vi "EnumDevicesEx2.vi"(5 "nLayerType":u32=1, 11 "error in (no error)":errorcluster caption="错误输入（无错误）") -> (4 "function return":i32, 6 "nDeviceNumReturn":u32, 8 "GigEDeviceArray":T4(array[cluster]), 10 "U3VDeviceArray":T3(array[cluster]), 12 "GenTLDevice":T1(array[cluster]), 15 "error out":errorcluster caption="错误输出")   [LabVIEW 2013, in "MvCameraControl.lvlib"]
uses:
  MvCameraControl.lvlib
  MvCameraPatch.dll
panel:
  in  "enSortMethod":T2(ring)
  in  "strManufacturerName":i8[](array[numeric])
  in  "U3VDevice":T5
  in  "GigEDevice":T6
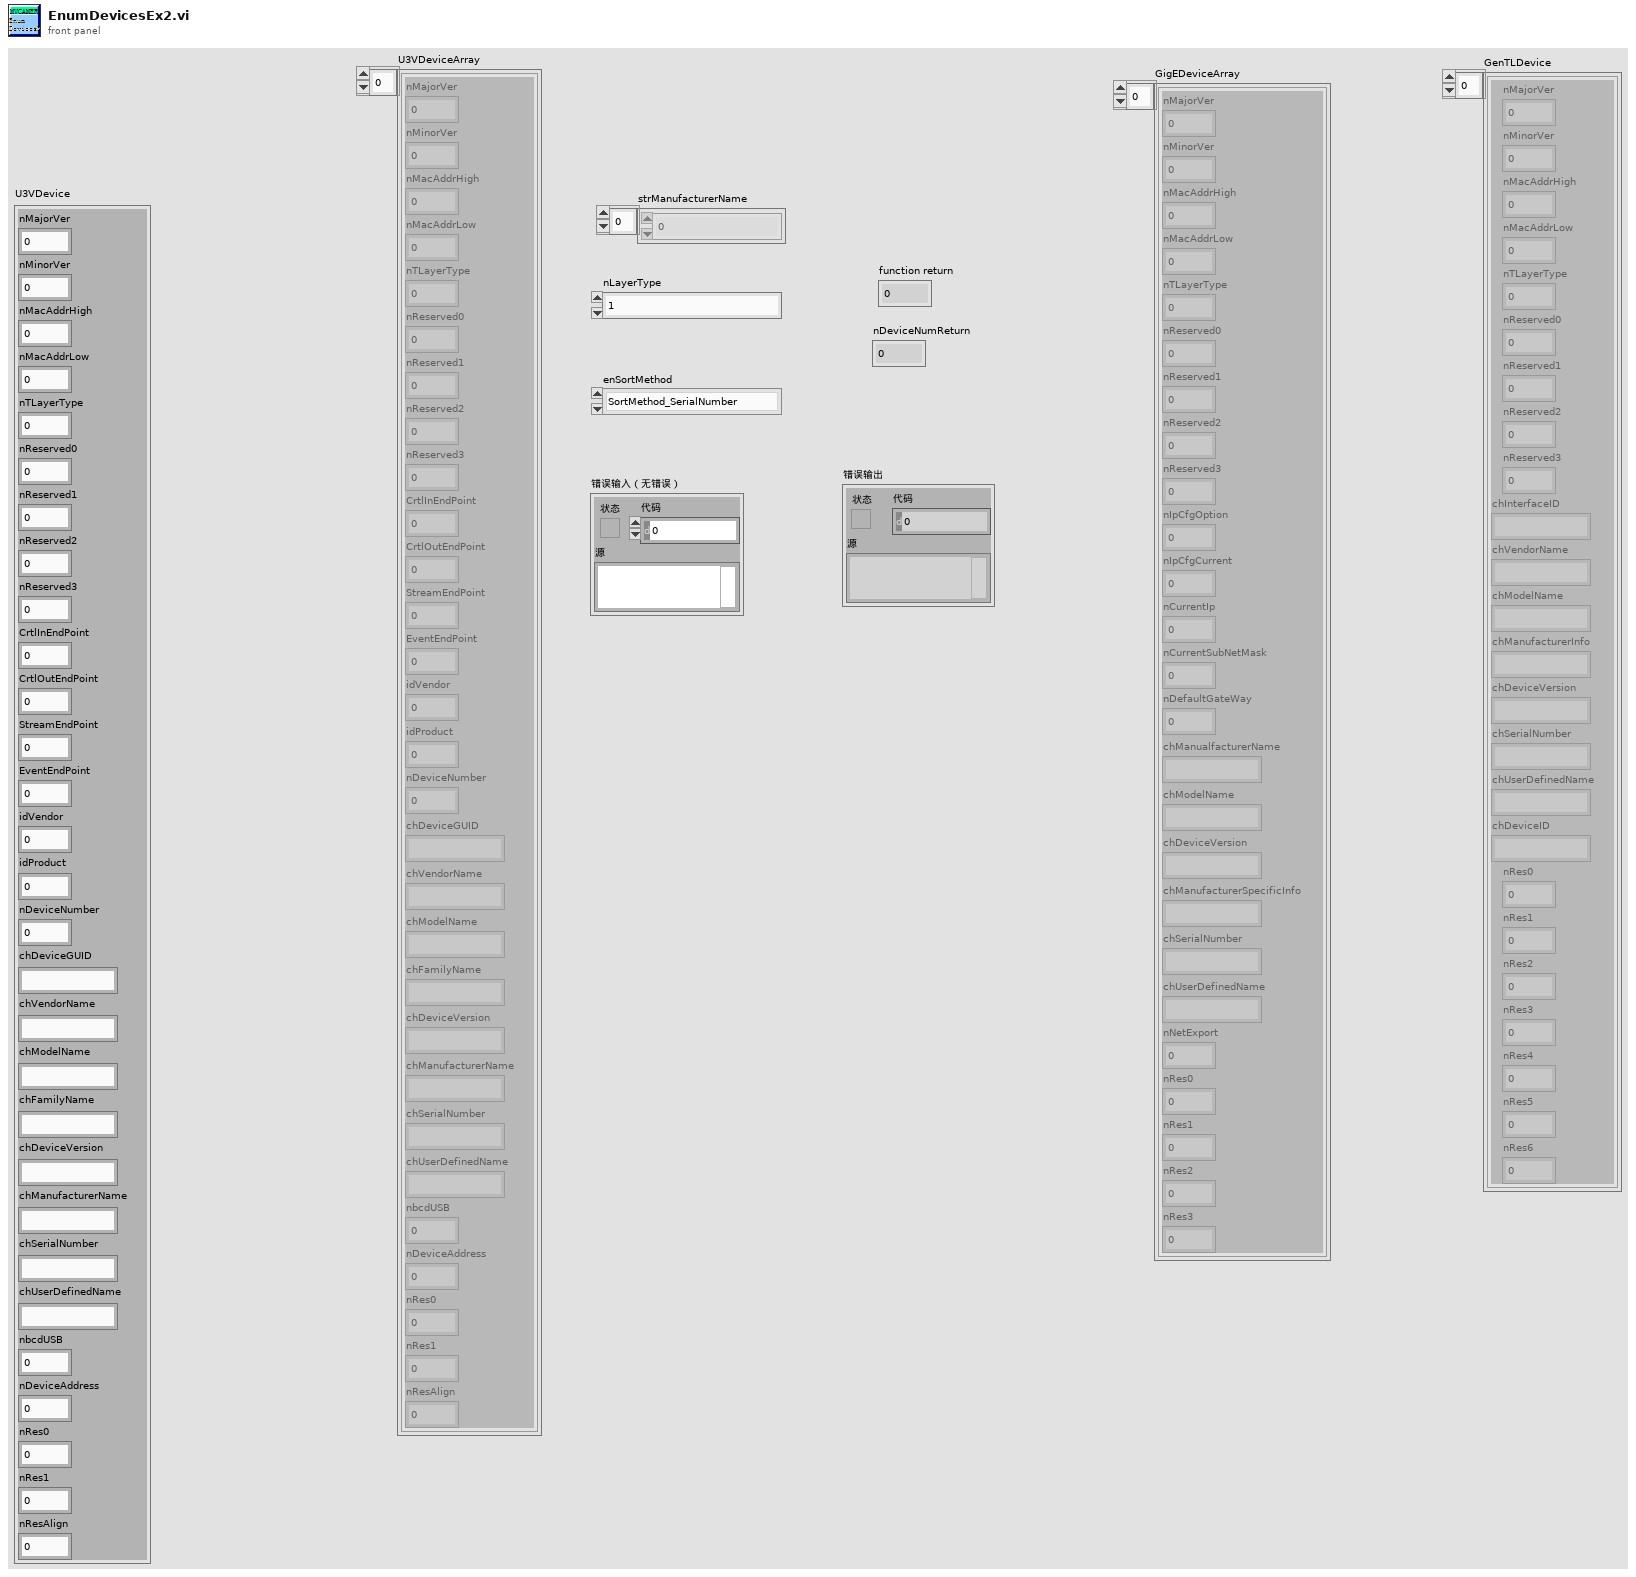
[diagram p1: front panel]
types:
  T1 = cluster{"nMajorVer":u16, "nMinorVer":u16, "nMacAddrHigh":u32, "nMacAddrLow":u32, "nTLayerType":u32, "nReserved0":u32, "nReserved1":u32, "nReserved2":u32, "nReserved3":u32, "chInterfaceID":string, "chVendorName":string, "chModelName":string, "chManufacturerInfo":string, "chDeviceVersion":string, "chSerialNumber":string, "chUserDefinedName":string, "chDeviceID":string, "nRes0":u32, "nRes1":u32, "nRes2":u32, "nRes3":u32, "nRes4":u32, "nRes5":u32, "nRes6":u32}[]
  T2 = enum16{"SortMethod_SerialNumber", "SortMethod_UserID", "SortMethod_CurrentIP_ASC", "SortMethod_CurrentIP_DESC"}
  T3 = cluster{"nMajorVer":u16, "nMinorVer":u16, "nMacAddrHigh":u32, "nMacAddrLow":u32, "nTLayerType":u32, "nReserved0":u32, "nReserved1":u32, "nReserved2":u32, "nReserved3":u32, "CrtlInEndPoint":u8, "CrtlOutEndPoint":u8, "StreamEndPoint":u8, "EventEndPoint":u8, "idVendor":u16, "idProduct":u16, "nDeviceNumber":u32, "chDeviceGUID":string, "chVendorName":string, "chModelName":string, "chFamilyName":string, "chDeviceVersion":string, "chManufacturerName":string, "chSerialNumber":string, "chUserDefinedName":string, "nbcdUSB":u32, "nDeviceAddress":u32, "nRes0":u32, "nRes1":u32, "nResAlign":u32}[]
  T4 = cluster{"nMajorVer":u16, "nMinorVer":u16, "nMacAddrHigh":u32, "nMacAddrLow":u32, "nTLayerType":u32, "nReserved0":u32, "nReserved1":u32, "nReserved2":u32, "nReserved3":u32, "nIpCfgOption":u32, "nIpCfgCurrent":u32, "nCurrentIp":u32, "nCurrentSubNetMask":u32, "nDefaultGateWay":u32, "chManualfacturerName":string, "chModelName":string, "chDeviceVersion":string, "chManufacturerSpecificInfo":string, "chSerialNumber":string, "chUserDefinedName":string, "nNetExport":u32, "nRes0":u32, "nRes1":u32, "nRes2":u32, "nRes3":u32}[]
  T5 = cluster{"nMajorVer":u16, "nMinorVer":u16, "nMacAddrHigh":u32, "nMacAddrLow":u32, "nTLayerType":u32, "nReserved0":u32, "nReserved1":u32, "nReserved2":u32, "nReserved3":u32, "CrtlInEndPoint":u8, "CrtlOutEndPoint":u8, "StreamEndPoint":u8, "EventEndPoint":u8, "idVendor":u16, "idProduct":u16, "nDeviceNumber":u32, "chDeviceGUID":string, "chVendorName":string, "chModelName":string, "chFamilyName":string, "chDeviceVersion":string, "chManufacturerName":string, "chSerialNumber":string, "chUserDefinedName":string, "nbcdUSB":u32, "nDeviceAddress":u32, "nRes0":u32, "nRes1":u32, "nResAlign":u32}
  T6 = cluster{"nMajorVer":u16, "nMinorVer":u16, "nMacAddrHigh":u32, "nMacAddrLow":u32, "nTLayerType":u32, "nReserved0":u32, "nReserved1":u32, "nReserved2":u32, "nReserved3":u32, "nIpCfgOption":u32, "nIpCfgCurrent":u32, "nCurrentIp":u32, "nCurrentSubNetMask":u32, "nDefaultGateWay":u32, "chManualfacturerName":string, "chModelName":string, "chDeviceVersion":string, "chManufacturerSpecificInfo":string, "chSerialNumber":string, "chUserDefinedName":string, "nNetExport":u32, "nRes0":u32, "nRes1":u32, "nRes2":u32, "nRes3":u32}
  T7 = cluster{"nMajorVer":u16, "nMinorVer":u16, "nMacAddrHigh":u32, "nMacAddrLow":u32, "nTLayerType":u32, "nReserved0":u32, "nReserved1":u32, "nReserved2":u32, "nReserved3":u32, "chInterfaceID":string, "chVendorName":string, "chModelName":string, "chManufacturerInfo":string, "chDeviceVersion":string, "chSerialNumber":string, "chUserDefinedName":string, "chDeviceID":string, "nRes0":u32, "nRes1":u32, "nRes2":u32, "nRes3":u32, "nRes4":u32, "nRes5":u32, "nRes6":u32}
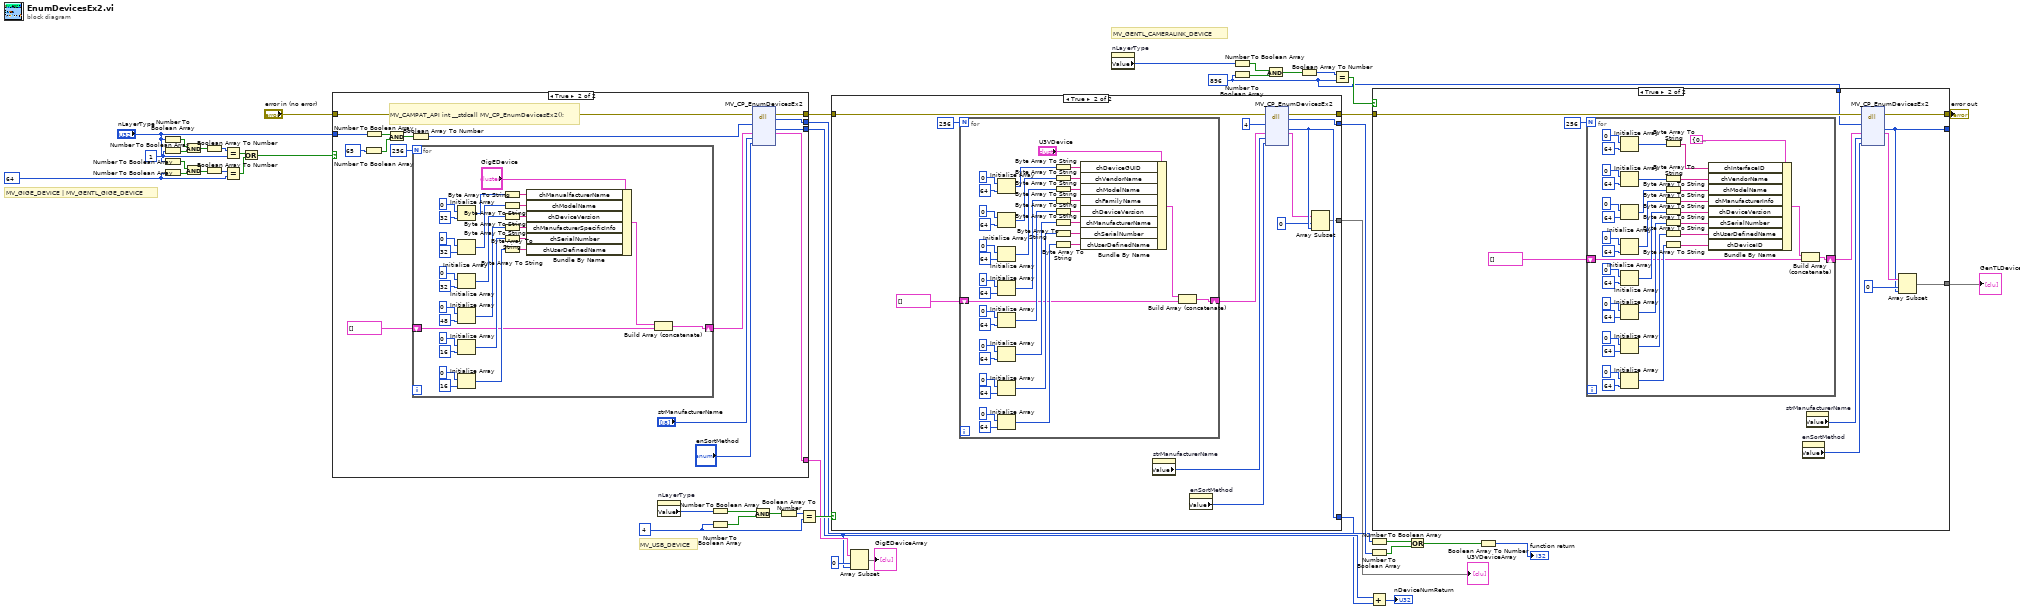
[diagram p0: block diagram]
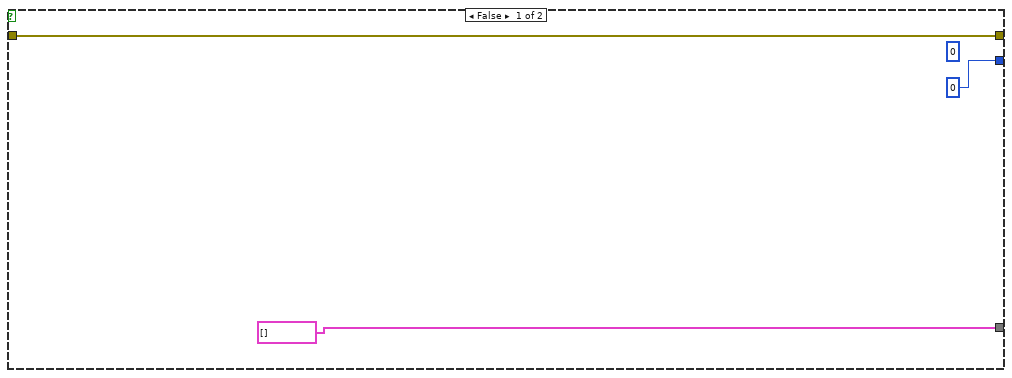
[diagram p2: hidden frame]
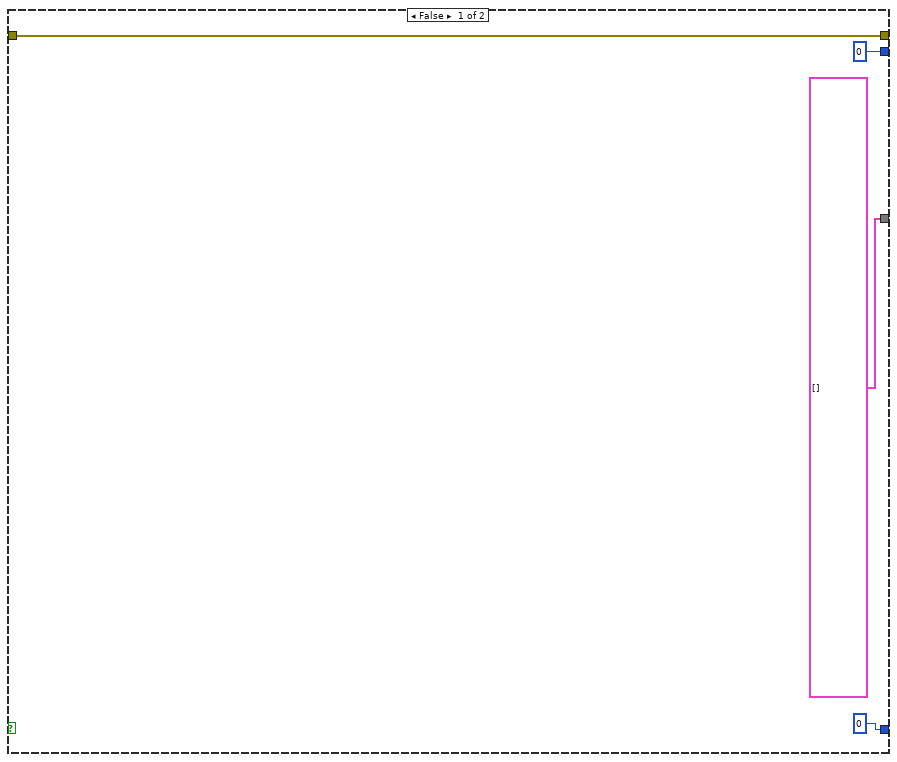
[diagram p3: hidden frame]
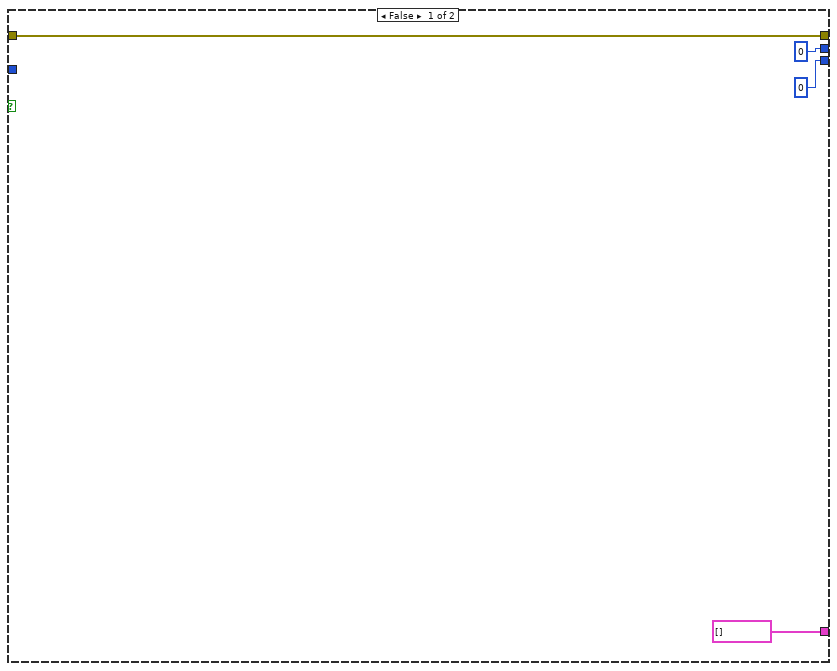
[diagram p4: hidden frame]
diagram:
  w2 = u32 896 ("数字")
  w17 = u32 64 ("数字")
  w36 = u32 4 ("数字")
  w42 = u32 1 ("数字")
  # "MV_GENTL_CAMERALINK_DEVICE"
  # "MV_USB_DEVICE"
  # "MV_GIGE_DEVICE | MV_GENTL_GIGE_DEVICE"
  n1 = Number To Boolean Array(number="nLayerType") -> (Boolean array=w46:bool[])
  n2 = Number To Boolean Array(number=w42) -> (Boolean array=w45:bool[])
  n3 = Number To Boolean Array(number="nLayerType") -> (Boolean array=w21:bool[])
  n4 = Number To Boolean Array(number=w17) -> (Boolean array=w20:bool[])
  n5 = And(x=w46, y=w45) -> (x .and. y?=w44:bool[])
  n6 = And(x=w21, y=w20) -> (x .and. y?=w19:bool[])
  n7 = Boolean Array To Number(Boolean array=w44) -> (number=w43:u32)
  n8 = Boolean Array To Number(Boolean array=w19) -> (number=w18:u32)
  n9 = Equal?(x=w43, y=w42) -> (x = y?=w15:bool)
  n10 = Equal?(x=w18, y=w17) -> (x = y?=w16:bool)
  n11 = Or(x=w15, y=w16) -> (x .or. y?=w14:bool)
  n12 = case shown="True" w14 {
    tunnel: [0 ("返回类型") w64] -> w32
    tunnel: [u32 0 ("nDeviceNumReturn") w63] -> w24
    tunnel: "error in (no error)" -> [w48 w62]
    tunnel: [w48 w61] -> w27
    tunnel: [T4 [] ("DeviceInfoArray") w59] -> w26
    tunnel: "nLayerType" -> [_ w52]
    frame False {
    }
    frame True {
      # "MV_CAMPAT_API int __stdcall MV_CP_EnumDevicesEx2();"
      n13 = Number To Boolean Array(number=u32 65 ("数字")) -> (Boolean array=w55:bool[])
      n14 = Number To Boolean Array(number=w52) -> (Boolean array=w56:bool[])
      n15 = And(x=w56, y=w55) -> (x .and. y?=w54:bool[])
      n16 = Boolean Array To Number(Boolean array=w54) -> (number=w51:u32)
      n17 = for {
        N: 256 -> [_]
        shift-right: [w69] -> w66
        shift-left: T4 [] -> [w67]
        n18 = Initialize Array(u8 0 ("元素"), 32 ("维数大小")) -> (w78:u8[])
        n19 = Initialize Array(u8 0 ("元素"), 32 ("维数大小")) -> (w81:u8[])
        n20 = Initialize Array(u8 0 ("元素"), 32 ("维数大小")) -> (w70:u8[])
        n21 = Initialize Array(u8 0 ("元素"), 48 ("维数大小")) -> (w75:u8[])
        n22 = Initialize Array(u8 0 ("元素"), 16 ("维数大小")) -> (w89:u8[])
        n23 = Initialize Array(u8 0 ("元素"), 16 ("维数大小")) -> (w86:u8[])
        n24 = Byte Array To String(unsigned byte array=w78) -> (string=w90:string)
        n25 = Byte Array To String(unsigned byte array=w81) -> (string=w91:string)
        n26 = Byte Array To String(unsigned byte array=w70) -> (string=w71:string)
        n27 = Byte Array To String(unsigned byte array=w75) -> (string=w92:string)
        n28 = Byte Array To String(unsigned byte array=w89) -> (string=w93:string)
        n29 = Byte Array To String(unsigned byte array=w86) -> (string=w94:string)
        n30 = Bundle By Name(cluster="GigEDevice", "chManualfacturerName"=w90, "chModelName"=w91, "chDeviceVersion"=w71, "chManufacturerSpecificInfo"=w92, "chSerialNumber"=w93, "chUserDefinedName"=w94) -> (w68:T6)
        n31 = Build Array (concatenate)(w68, w67) -> (w69:T4)
      }
      n32 = dll-call lib="MvCameraPatch.dll" fn="MV_CP_EnumDevicesEx2"(error in=w62, "nLayerType"=w51, "DeviceInfoArray"=w66, "strManufacturerName"="strManufacturerName", "enSortMethod"="enSortMethod") -> (error out=w61:errorcluster, "返回类型"=w64:i32, "nDeviceNumReturn"=w63:u32, "DeviceInfoArray"=w59:T4)  [unwired: 6 in, 1 out]
    }
  }
  n33 = property on="nLayerType" class="DigNum (strict)"() -> ("Value"=w8:u32)  [unwired: 2 in, 2 out]
  n34 = Number To Boolean Array(number=w8) -> (Boolean array=w40:bool[])
  n35 = Number To Boolean Array(number=w36) -> (Boolean array=w39:bool[])
  n36 = And(x=w40, y=w39) -> (x .and. y?=w38:bool[])
  n37 = Boolean Array To Number(Boolean array=w38) -> (number=w37:u32)
  n38 = Equal?(x=w37, y=w36) -> (x = y?=w35:bool)
  n39 = case shown="True" w35 {
    tunnel: [u32 0 ("nDeviceNumReturn") w110] -> w22
    tunnel: [0 ("返回类型") w109] -> w33
    tunnel: w27 -> [w96 w108]
    tunnel: [w96 w107] -> w7
    tunnel: [T3 [] w99] -> w3
    frame False {
    }
    frame True {
      n40 = for {
        N: 256 -> [_]
        shift-right: [w112] -> w105
        shift-left: T3 [] -> [w114]
        n41 = Initialize Array(u8 0 ("元素"), 64 ("维数大小")) -> (w118:u8[])
        n42 = Initialize Array(u8 0 ("元素"), 64 ("维数大小")) -> (w122:u8[])
        n43 = Initialize Array(u8 0 ("元素"), 64 ("维数大小")) -> (w125:u8[])
        n44 = Initialize Array(u8 0 ("元素"), 64 ("维数大小")) -> (w128:u8[])
        n45 = Initialize Array(u8 0 ("元素"), 64 ("维数大小")) -> (w131:u8[])
        n46 = Initialize Array(u8 0 ("元素"), 64 ("维数大小")) -> (w134:u8[])
        n47 = Initialize Array(u8 0 ("元素"), 64 ("维数大小")) -> (w141:u8[])
        n48 = Initialize Array(u8 0 ("元素"), 64 ("维数大小")) -> (w146:u8[])
        n49 = Byte Array To String(unsigned byte array=w118) -> (string=w119:string)
        n50 = Byte Array To String(unsigned byte array=w122) -> (string=w135:string)
        n51 = Byte Array To String(unsigned byte array=w125) -> (string=w136:string)
        n52 = Byte Array To String(unsigned byte array=w128) -> (string=w137:string)
        n53 = Byte Array To String(unsigned byte array=w131) -> (string=w138:string)
        n54 = Byte Array To String(unsigned byte array=w134) -> (string=w142:string)
        n55 = Byte Array To String(unsigned byte array=w141) -> (string=w143:string)
        n56 = Byte Array To String(unsigned byte array=w146) -> (string=w147:string)
        n57 = Bundle By Name(cluster="U3VDevice", "chDeviceGUID"=w119, "chVendorName"=w135, "chModelName"=w136, "chFamilyName"=w137, "chDeviceVersion"=w138, "chManufacturerName"=w142, "chSerialNumber"=w143, "chUserDefinedName"=w147) -> (w113:T5)
        n58 = Build Array (concatenate)(w113, w114) -> (w112:T3)
      }
      n59 = property on="strManufacturerName" class="Arr (strict)"() -> ("Value"=w103:i8[])  [unwired: 2 in, 2 out]
      n60 = property on="enSortMethod" class="Enum (strict)"() -> ("Value"=w102:T2)  [unwired: 2 in, 2 out]
      n61 = dll-call lib="MvCameraPatch.dll" fn="MV_CP_EnumDevicesEx2"(error in=w108, "nLayerType"=u32 4, "DeviceInfoArray"=w105, "strManufacturerName"=w103, "enSortMethod"=w102) -> (error out=w107:errorcluster, "返回类型"=w109:i32, "nDeviceNumReturn"=w110:u32, "DeviceInfoArray"=w101:T3)  [unwired: 6 in, 1 out]
      n62 = Array Subset(array=w101, index=0, length=w110) -> (w99:T3)
    }
  }
  "U3VDeviceArray" <- w3
  n63 = Array Subset(array=w26, index=0, length=w24) -> (→"GigEDeviceArray":T4)
  n64 = property on="nLayerType" class="DigNum (strict)"() -> ("Value"=w4:u32)  [unwired: 2 in, 2 out]
  n65 = Number To Boolean Array(number=w4) -> (Boolean array=w12:bool[])
  n66 = Number To Boolean Array(number=w2) -> (Boolean array=w11:bool[])
  n67 = And(x=w12, y=w11) -> (x .and. y?=w10:bool[])
  n68 = Boolean Array To Number(Boolean array=w10) -> (number=w9:u32)
  n69 = Equal?(x=w9, y=w2) -> (x = y?=w5:bool)
  n70 = Add(x=w24, y=w22) -> (x+y=→"nDeviceNumReturn":u32)
  n71 = Number To Boolean Array(number=w32) -> (Boolean array=w31:bool[])
  n72 = Number To Boolean Array(number=w33) -> (Boolean array=w30:bool[])
  n73 = case shown="True" w5 {
    tunnel: [u32 0 ("nDeviceNumReturn") w153] -> _
    tunnel: w7 -> [w149 w162]
    tunnel: [w149 w161] -> w6
    tunnel: w2 -> [_ w152]
    tunnel: [T1 [] w151] -> w1
    frame False {
      (unwired) 0 ("返回类型")
    }
    frame True {
      n74 = for {
        N: 256 -> [_]
        shift-right: [w166] -> w159
        shift-left: T1 [] -> [w168]
        n75 = Initialize Array(u8 0 ("元素"), 64 ("维数大小")) -> (w171:u8[])
        n76 = Initialize Array(u8 0 ("元素"), 64 ("维数大小")) -> (w175:u8[])
        n77 = Initialize Array(u8 0 ("元素"), 64 ("维数大小")) -> (w178:u8[])
        n78 = Initialize Array(u8 0 ("元素"), 64 ("维数大小")) -> (w181:u8[])
        n79 = Initialize Array(u8 0 ("元素"), 64 ("维数大小")) -> (w184:u8[])
        n80 = Initialize Array(u8 0 ("元素"), 64 ("维数大小")) -> (w187:u8[])
        n81 = Initialize Array(u8 0 ("元素"), 64 ("维数大小")) -> (w193:u8[])
        n82 = Initialize Array(u8 0 ("元素"), 64 ("维数大小")) -> (w197:u8[])
        n83 = Byte Array To String(unsigned byte array=w171) -> (string=w172:string)
        n84 = Byte Array To String(unsigned byte array=w175) -> (string=w188:string)
        n85 = Byte Array To String(unsigned byte array=w178) -> (string=w189:string)
        n86 = Byte Array To String(unsigned byte array=w181) -> (string=w163:string)
        n87 = Byte Array To String(unsigned byte array=w184) -> (string=w190:string)
        n88 = Byte Array To String(unsigned byte array=w187) -> (string=w164:string)
        n89 = Byte Array To String(unsigned byte array=w193) -> (string=w194:string)
        n90 = Byte Array To String(unsigned byte array=w197) -> (string=w198:string)
        n91 = Bundle By Name(cluster=T7 {"nMajorVer"=0, "nMinorVer"=0, "nMacAddrHigh"=0, "nMacAddrLow"=0, "nTLayerType"=0, "nReserved0"=0, "nReserved1"=0, "nReserved2"=0, "nReserved3"=0, "chInterfaceID"="", "chVendorName"="", "chModelName"="", "chManufacturerInfo"="", "chDeviceVersion"="", "chSerialNumber"="", "chUserDefinedName"="", "chDeviceID"="", "nRes0"=0, "nRes1"=0, "nRes2"=0, "nRes3"=0, "nRes4"=0, "nRes5"=0, "nRes6"=0} ("GenTLCMLDevice"), "chInterfaceID"=w172, "chVendorName"=w188, "chModelName"=w189, "chManufacturerInfo"=w163, "chDeviceVersion"=w190, "chSerialNumber"=w164, "chUserDefinedName"=w194, "chDeviceID"=w198) -> (w167:T7)
        n92 = Build Array (concatenate)(w167, w168) -> (w166:T1)
      }
      n93 = property on="enSortMethod" class="Enum (strict)"() -> ("Value"=w156:T2)  [unwired: 2 in, 2 out]
      n94 = property on="strManufacturerName" class="Arr (strict)"() -> ("Value"=w157:i8[])  [unwired: 2 in, 2 out]
      n95 = dll-call lib="MvCameraPatch.dll" fn="MV_CP_EnumDevicesEx2"(error in=w162, "nLayerType"=w152, "DeviceInfoArray"=w159, "strManufacturerName"=w157, "enSortMethod"=w156) -> (error out=w161:errorcluster, "nDeviceNumReturn"=w153:u32, "DeviceInfoArray"=w154:T1)  [unwired: 7 in, 1 out]
      n96 = Array Subset(array=w154, index=0, length=w153) -> (w151:T1)
    }
  }
  "error out" <- w6
  "GenTLDevice" <- w1
  n97 = Or(x=w31, y=w30) -> (x .or. y?=w29:bool[])
  n98 = Boolean Array To Number(Boolean array=w29) -> (number=→"function return":u32)
